vi "keepalive.vi"() -> ()   [LabVIEW 2017]
doc: "Illustrates how to configure keep-alive messages and send them in blocking and non-blocking mode."
uses:
  libssh2/libssh2_session_handshake_tcp.vi
  libssh2/libssh2_init_default.vi
  libssh2/libssh2_session_init_ex.vi
  <vilib>/Utility/tcp.llb/TCP Get Raw Net Object.vi
  libssh2/libssh2_session_handshake_socket.vi
  libssh2/libssh2_userauth_password_ex.vi
  libssh2/libssh2.lvlib
panel:
  in  "want reply":bool=TRUE
  in  "interval (0 = disabled)":u32=10
  out "seconds to next":i32
  in  "Stop Button":bool
  in  "password":string
  in  "username":string
  out "error out":errorcluster
  in  "hostname":string="localhost"
  # "The number of seconds to wait between keep-alive messages.\nlibssh2 will treat an interval of 1 as 2 for \"busy-loop reasons\"."
  # "Configure whether we expect a reply to the keep-alive message.\nNote: the server is not required to send a reply, even when this option is enabled."
  # "Indicates how many seconds we should wait before the next keep-alive message is sent.\nNote: Keep-alive is successful as long as no error is returned."
  # "Press the stop button to stop sending keep-alive messages."
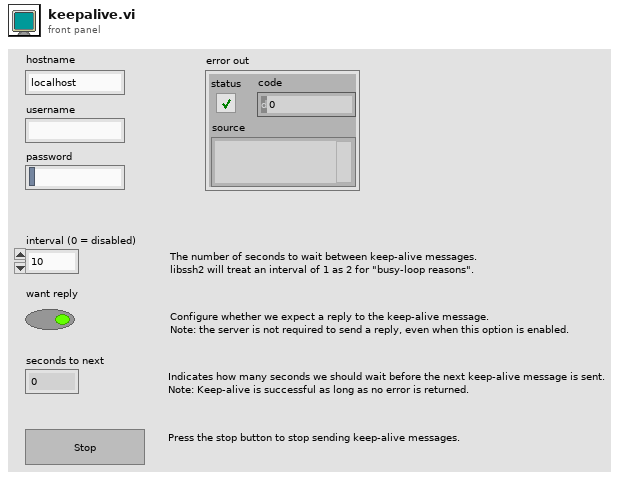
[diagram p1: front panel]
types:
  T1 = typedef "libssh2.lvlib/Session Refnum.ctl" = refnum<k1>
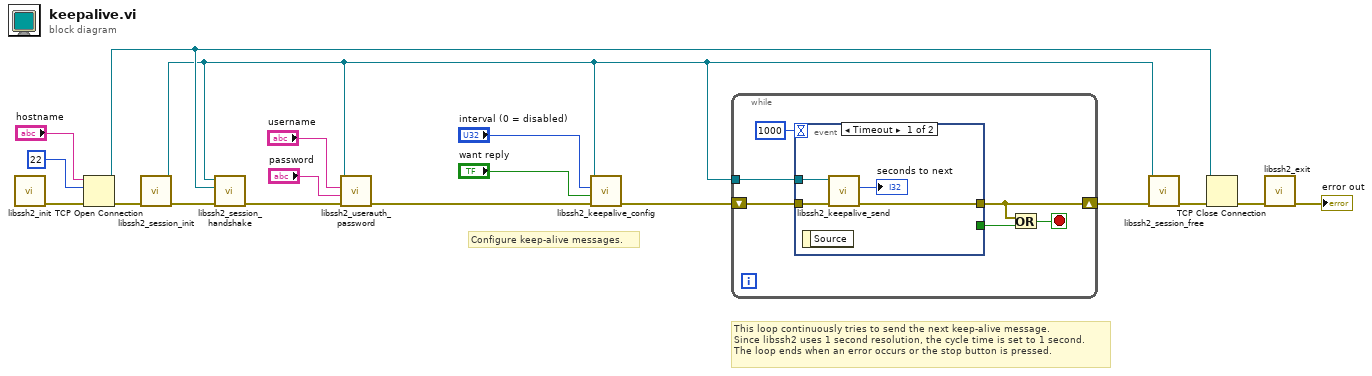
[diagram p0: block diagram]
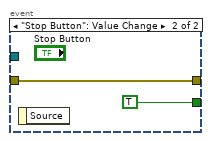
[diagram p2: hidden frame]
diagram:
  # "This loop continuously tries to send the next keep-alive message.\nSince libssh2 uses 1 second resolution, the cycle time is set to 1 second.\nThe loop ends when an error occurs or the stop button is pressed."
  # "Configure keep-alive messages."
  n1 = call-poly "libssh2_init.vi"() -> ("error out"=w5:errorcluster)  [unwired: 11 in]
  n2 = TCP Open Connection(address="hostname", remote port or service name=u16 22, error in (no error)=w5) -> (connection ID=w12:refnum<k5>, error out=w6:errorcluster)  [unwired: 2 in]
  n3 = call "libssh2_session_init.vi"("error in (no error)"=w6) -> ("error out"=w7:errorcluster, "session"=w9:T1)  [unwired: 9 in]
  n4 = call-poly "libssh2_session_handshake.vi"("error in (no error)"=w7, "tcp connection"=w12, "session"=w9) -> ("error out"=w4:errorcluster)  [unwired: 8 in]
  n5 = call "libssh2_userauth_password.vi"("error in (no error)"=w4, "password"="password", "username"="username", "session"=w9) -> ("error out"=w3:errorcluster)  [unwired: 7 in]
  n6 = call "libssh2_keepalive_config.vi"("error in (no error)"=w3, "want reply (F)"="want reply", "interval (0 = disabled)"="interval (0 = disabled)", "session"=w9) -> ("error out"=w2:errorcluster)  [unwired: 7 in]
  n7 = while {
    tunnel: w9 -> [w23]
    shift-right: [w22] -> w10
    shift-left: w2 -> [w24]
    stop <- w20 stop-if-true
    n8 = event shown="[0] Timeout" {
      selector: _ -> [_ _]
      dyn-events: _ -> [_ _]
      timeout: 1000 -> [_ _]
      tunnel: [w27 w30] -> w22
      tunnel: w24 -> [w28 w30]
      tunnel: w23 -> [w26 _]
      tunnel: [_ TRUE] -> w21
      event Timeout {
        n9 = event-data() -> ()  [unwired: 1 in, 1 out]
        n10 = call "libssh2_keepalive_send.vi"("error in (no error)"=w28, "session"=w26) -> ("error out"=w27:errorcluster, "seconds to next"=→"seconds to next":i32)  [unwired: 8 in]
      }
      event "Stop Button": Value Change {
        n11 = event-data() -> ()  [unwired: 1 in, 1 out]
      }
    }
    n12 = Or(x=w22, y=w21) -> (x .or. y?=w20:bool)
  }
  n13 = call "libssh2_session_free.vi"("error in (no error)"=w10, "session"=w9) -> ("error out"=w18:errorcluster)  [unwired: 9 in]
  n14 = TCP Close Connection(connection ID=w12, error in (no error)=w18) -> (error out=w13:errorcluster)  [unwired: 1 in, 1 out]
  n15 = call "libssh2_exit.vi"("error in (no error)"=w13) -> ("error out"=→"error out":errorcluster)  [unwired: 10 in]
